vi "Valve State.vi"() -> ()   [LabVIEW 2012, in "Temperature Controller.lvclass"]
uses:
  Temperature Controller.lvclass
panel:
  in  "Est position (%)":dbl
  out "Needle Valve open/close rate (ms)":dbl=66000.0
  out "Needle Valve Timestamp":u32
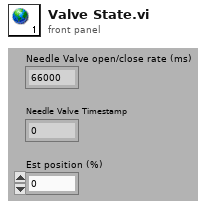
[diagram p1: front panel]
diagram:
